vi "HMI_Cocina.vi"() -> ()   [LabVIEW 2023]
uses:
  <vilib>/Instr/_visa.llb/VISA Configure Serial Port (Instr).vi
panel:
  out "Ingresos":string
  out "read buffer":string
  in  "stop":bool
  in  "Pedido a despachar":i32(listbox)
  out "cntPlato3":dbl
  out "cntPlato2":dbl
  out "cntPlato1":dbl
  out "cntPlato0":dbl
  in  "VISA resource name":refnum<visa-resource-name>
  in  "Enviar":bool
  # "ENTRADA DE PEDIDOS"
  # "ORDEN        CANTIDAD"
  # "Salchipapa\n\nChaulafan\n\nEncebollado\n\nGuatita"
  # "DESPACHO DE PEDIDO"
  # "$"
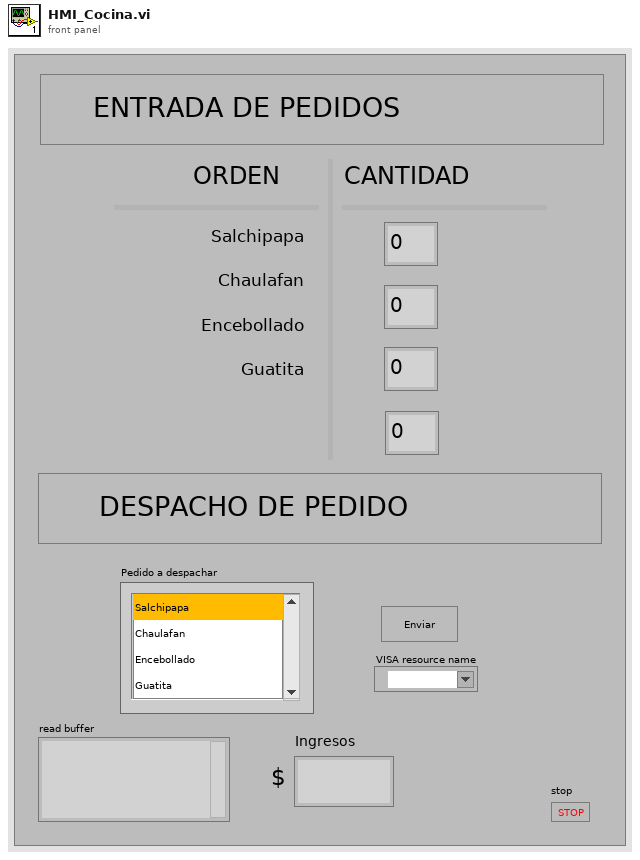
[diagram p1: front panel]
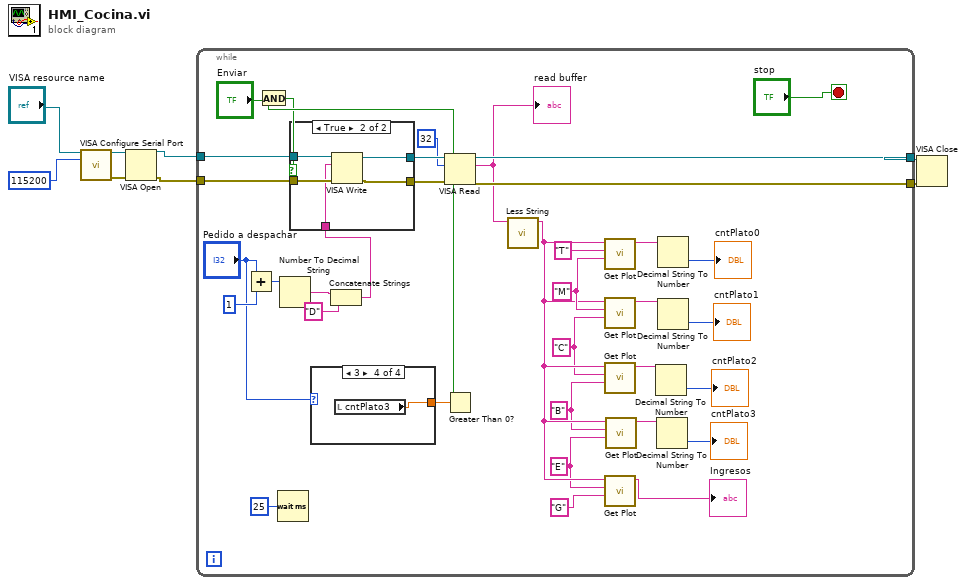
[diagram p0: block diagram]
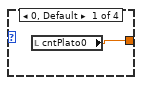
[diagram p2: hidden frame]
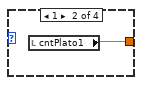
[diagram p3: hidden frame]
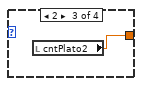
[diagram p4: hidden frame]
diagram:
  n1 = call-poly "VISA Configure Serial Port"("VISA resource name"="VISA resource name", "baud rate (9600)"=u32 115200) -> ("VISA resource name out"=w6:refnum<visa-resource-name>, "error out"=w7:errorcluster)  [unwired: 12 in]
  n2 = VISA Open(error in (no error)=w7, VISA resource name=w6) -> (VISA resource name=w5:refnum<visa-resource-name>, error out=w4:errorcluster)  [unwired: 3 in]
  n3 = while {
    tunnel: w5 -> [w44]
    tunnel: w4 -> [w43]
    tunnel: [w40] -> w2
    tunnel: [w39] -> w1
    stop <- "stop" stop-if-true
    w32 = "E" ("Start")
    w33 = "B" ("Start")
    w34 = "C" ("Start")
    w36 = "M" ("Start")
    n4 = Add(x="Pedido a despachar", y=1) -> (x+y=w14:i32)
    n5 = Wait (ms)(milliseconds to wait=u32 25) -> ()  [unwired: 1 out]
    n6 = Number To Decimal String(number=w14) -> (decimal integer string=w18:string)  [unwired: 1 in]
    n7 = case shown="3" "Pedido a despachar" {
      tunnel: [w45 w46 w47 w48] -> w12
      frame 0, Default {
        n8 = local read "cntPlato0"() -> (w45:dbl)
      }
      frame 1 {
        n9 = local read "cntPlato1"() -> (w46:dbl)
      }
      frame 2 {
        n10 = local read "cntPlato2"() -> (w47:dbl)
      }
      frame 3 {
        n11 = local read "cntPlato3"() -> (w48:dbl)
      }
    }
    n12 = Concatenate Strings(w18, "D" ("string")) -> (w16:string)
    n13 = Greater Than 0?(x=w12) -> (x > 0?=w10:bool)
    n14 = And(x="Enviar", y=w10) -> (x .and. y?=w9:bool)
    n15 = case shown="True" w9 {
      tunnel: w44 -> [w50 w55]
      tunnel: w43 -> [w49 w54]
      tunnel: [w50 w53] -> w42
      tunnel: [w49 w52] -> w41
      tunnel: w16 -> [_ w51]
      frame False {
      }
      frame True {
        n16 = VISA Write(VISA resource name=w55, write buffer=w51, error in (no error)=w54) -> (VISA resource name out=w53:refnum<visa-resource-name>, error out=w52:errorcluster)  [unwired: 1 out]
      }
    }
    n17 = VISA Read(VISA resource name=w42, byte count=u32 32, error in (no error)=w41) -> (VISA resource name out=w39:refnum<visa-resource-name>, read buffer=w38:string, error out=w40:errorcluster)  [unwired: 1 out]
    "read buffer" <- w38
    n18 = call "Less String.vi"("Input String"=w38) -> ("Out String"=w35:string)  [unwired: 10 in]
    n19 = call "Get Plot.vi"("Stop"=w36, "Start"="T", "Input String"=w35) -> ("Out String"=w30:string)  [unwired: 8 in]
    n20 = call "Get Plot.vi"("Stop"=w34, "Start"=w36, "Input String"=w35) -> ("Out String"=w29:string)  [unwired: 8 in]
    n21 = call "Get Plot.vi"("Stop"=w33, "Start"=w34, "Input String"=w35) -> ("Out String"=w28:string)  [unwired: 8 in]
    n22 = call "Get Plot.vi"("Stop"="G" ("Start"), "Start"=w32, "Input String"=w35) -> ("Out String"=→"Ingresos":string)  [unwired: 8 in]
    n23 = call "Get Plot.vi"("Stop"=w32, "Start"=w33, "Input String"=w35) -> ("Out String"=w27:string)  [unwired: 8 in]
    n24 = Decimal String To Number(string=w28) -> (number=→"cntPlato2":i32)  [unwired: 2 in, 1 out]
    n25 = Decimal String To Number(string=w27) -> (number=→"cntPlato3":i32)  [unwired: 2 in, 1 out]
    n26 = Decimal String To Number(string=w30) -> (number=→"cntPlato0":i32)  [unwired: 2 in, 1 out]
    n27 = Decimal String To Number(string=w29) -> (number=→"cntPlato1":i32)  [unwired: 2 in, 1 out]
  }
  n28 = VISA Close(VISA resource name=w1, error in (no error)=w2) -> ()  [unwired: 1 out]
